vi "Cash String to Data.vi"(11 "Cash Data String":string) -> (2 "Cash Data Array":T1(array[cluster]), 3 "Cash Player Name Array":string[](array[string]))   [LabVIEW 2021]
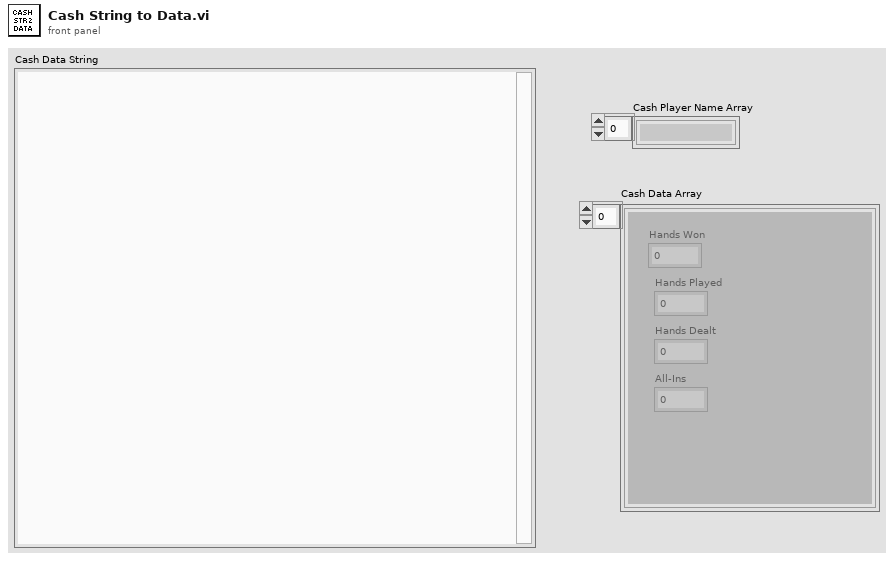
[diagram p1: front panel]
types:
  T1 = cluster{"Hands Won":u32, "Hands Played":u32, "Hands Dealt":u32, "All-Ins":u32}[]
  T2 = cluster{"Numeric":i32, "Numeric":i32, "Numeric":i32, "Numeric":i32}
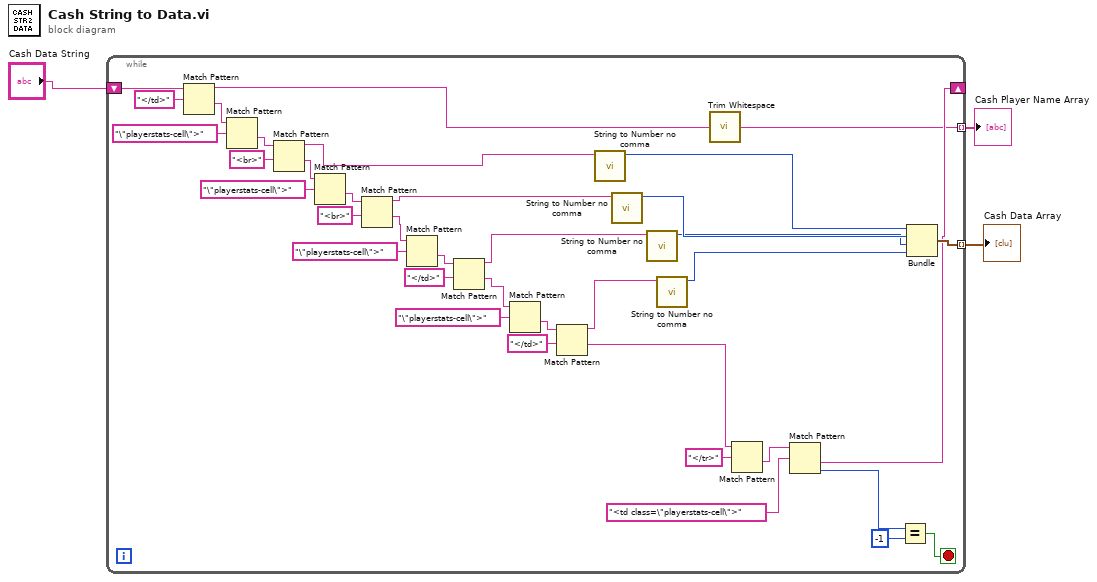
[diagram p0: block diagram]
diagram:
  n1 = while {
    shift-right: [w6] -> _
    shift-left: "Cash Data String" -> [w40]
    tunnel: [w4] -> w3 mode=indexing
    tunnel: [w18] -> w1 mode=indexing
    stop <- w20 stop-if-true
    n2 = Match Pattern(string=w40, regular expression="</td>") -> (before substring=w19:string, after substring=w38:string)  [unwired: 1 in, 2 out]
    n3 = Match Pattern(string=w38, regular expression="\"playerstats-cell\">") -> (after substring=w36:string)  [unwired: 1 in, 3 out]
    n4 = Match Pattern(string=w36, regular expression="<br>") -> (before substring=w17:string, after substring=w31:string)  [unwired: 1 in, 2 out]
    n5 = Match Pattern(string=w31, regular expression="\"playerstats-cell\">") -> (after substring=w33:string)  [unwired: 1 in, 3 out]
    n6 = Match Pattern(string=w33, regular expression="<br>") -> (before substring=w14:string, after substring=w28:string)  [unwired: 1 in, 2 out]
    n7 = Match Pattern(string=w28, regular expression="\"playerstats-cell\">") -> (after substring=w30:string)  [unwired: 1 in, 3 out]
    n8 = Match Pattern(string=w30, regular expression="</td>") -> (before substring=w12:string, after substring=w23:string)  [unwired: 1 in, 2 out]
    n9 = Match Pattern(string=w23, regular expression="\"playerstats-cell\">") -> (after substring=w24:string)  [unwired: 1 in, 3 out]
    n10 = Match Pattern(string=w24, regular expression="</td>") -> (before substring=w10:string, after substring=w15:string)  [unwired: 1 in, 2 out]
    n11 = call "String to Number no comma.vi"("Number String"=w17) -> ("Numeric"=w16:i32)  [unwired: 10 in]
    n12 = call "String to Number no comma.vi"("Number String"=w14) -> ("Numeric"=w13:i32)  [unwired: 10 in]
    n13 = call "String to Number no comma.vi"("Number String"=w12) -> ("Numeric"=w11:i32)  [unwired: 10 in]
    n14 = call "String to Number no comma.vi"("Number String"=w10) -> ("Numeric"=w9:i32)  [unwired: 10 in]
    n15 = call <vilib>:"Trim Whitespace.vi"("string"=w19) -> ("trimmed string"=w4:string)  [unwired: 1 in]
    n16 = Match Pattern(string=w15, regular expression="</tr>") -> (after substring=w8:string)  [unwired: 1 in, 3 out]
    n17 = Match Pattern(string=w8, regular expression="<td class=\"playerstats-cell\">") -> (after substring=w6:string, offset past match=w5:i32)  [unwired: 1 in, 2 out]
    n18 = Equal?(x=w5, y=-1) -> (x = y?=w20:bool)
    n19 = Bundle("Numeric"=w16, "Numeric"=w13, "Numeric"=w11, "Numeric"=w9) -> (w18:T2)  [unwired: 1 in]
  }
  "Cash Player Name Array" <- w3
  "Cash Data Array" <- w1
